vi "Class to Variant.vi"(8 "error in (no error)":errorcluster, 11 "LabVIEW Build in":refnum<class "LabVIEW Build.lvclass">) -> (0 "error out":errorcluster, 1 "Display":string, 2 "Data":variant, 3 "LabVIEW Build out":refnum<class "LabVIEW Build.lvclass">)   [LabVIEW 2014, in "LabVIEW Build.lvclass"]
uses:
  LabVIEW Build.lvclass
  LabVIEW Build.lvclass/LabVIEW Build.ctl
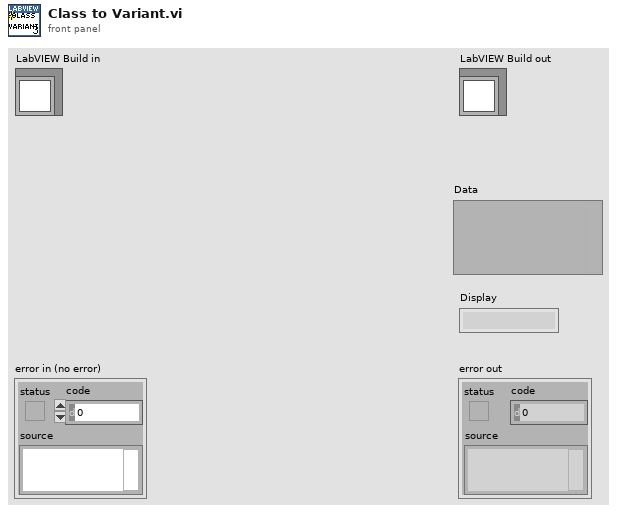
[diagram p1: front panel]
types:
  T1 = typedef "LabVIEW Build - STYP.ctl" = cluster{"Executor_Number":string, "Workspace_Path":string, "Build_Spec":string, "Project_Path":string, "Auto_Version_Increment":bool}
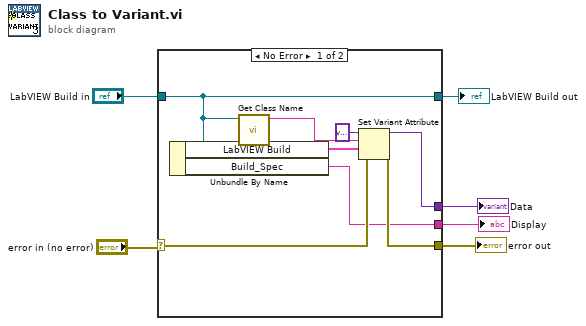
[diagram p0: block diagram]
diagram:
  n1 = case shown="No Error" "error in (no error)" {
    selector: "error in (no error)" -> [w11 w15]
    tunnel: "LabVIEW Build in" -> [w9 w16]
    tunnel: [w9 w16] -> w4
    tunnel: [w12 _] -> w3
    tunnel: [w10 w15] -> w2
    tunnel: [w7 _] -> w1
    frame No Error {
      n2 = Unbundle By Name(w9) -> ("LabVIEW Build"=w14:T1, "Build_Spec"=w7:string)
      n3 = call "Get Class Name.vi"("lvclass"=w9) -> ("Class Name"=w8:string)  [unwired: 10 in]
      n4 = Set Variant Attribute(Variant=variant ("variant"), name=w8, value=w14, error in=w11) -> (Variant out=w12:variant, error out=w10:errorcluster)  [unwired: 1 out]
    }
    frame Error {
    }
  }
  "error out" <- w2
  "LabVIEW Build out" <- w4
  "Data" <- w3
  "Display" <- w1
